vi "FRCts20_Backend_AdministratorInterface.vi"() -> ()   [LabVIEW 2014, in "FRCts20_Backend_TestCode.lvlib"]
uses:
  FRCts20_Backend_TestCode.lvlib
  FRCts20_Backend_Engine.lvlib
  FRCts20_Backend_FGVOperation.ctl
  FRCts20_Backend_DequeueDataOperations.ctl
  FRCts20_Backend_WebMethods.lvlib
  <vilib>/Utility/error.llb/DialogType.ctl
  FRCts20_Backend_IssueDfn.ctl
  FRCts20_Backend_Controls.lvlib
  FRCts20_Backend_TeamDfn.ctl
  FRCts20_Backend_PercTeams.ctl
  FRCts20_Backend_ResDayTotals.ctl
  FRCts20_Backend_ResQuadTotals.ctl
  FRCts20_Backend_OpenQuadTotals.ctl
  FRCts20_Backend_TeamList.ctl
  FRCts20_Backend_IssueTeamList.ctl
  FRCts20_Backend_Team_Info.ctl
  FRCts20_Backend_Note.ctl
  FRCts20_Backend_Note_list.ctl
  FRCts20_Backend_request_info.ctl
panel:
  in  "Tab Control":T1(tab)
  out "Status?":string
  in  "Add Team":bool
  in  "Add Team":T2
  in  "Exit":bool
  in  "Team Number?":u16
  in  "Get Team":bool
  out "Get Team":T2
  out "Key (Return)":string
  out "Message Value (Return)":string
  out "Message (Return)":string
  in  "DeQueue Data":bool
  in  "Key":string
  in  "Message Value":string
  in  "Message Name":string
  in  "Send Meassage":bool
  out "IssueTeamList":T4
  in  "Get Issue Team List":bool
  in  "Get Team List":bool
  out "TeamList":T9
  in  "Get Stats":bool
  out "Issues.Open.QuadTotals":T10
  out "Issues.Open.Total":u16
  out "SoftwareUsage.PercTeams":T11
  out "Issues.Resolved.Total":u16
  out "Issues.Resolved.AvgTimeRes":dbl
  out "Issues.Resolved.QuadTotals":T12
  out "Issues.Resolved.DayTotals":T13
  in  "Exit Run-Time  2":bool
  in  "Edit Exit":bool
  in  "Set Dates":bool
  in  "Competition Start Date":timestamp
  in  "Path to GenerateStats.vi":path=path "C:/FRC Team Service/source/VI Source/FRCts20_Backend_GenerateStats.vi"
  out "Complete?":bool
  # "Run-Time Tools"
  # "Run-Time Tools"
  # "Edit-Time Tools"
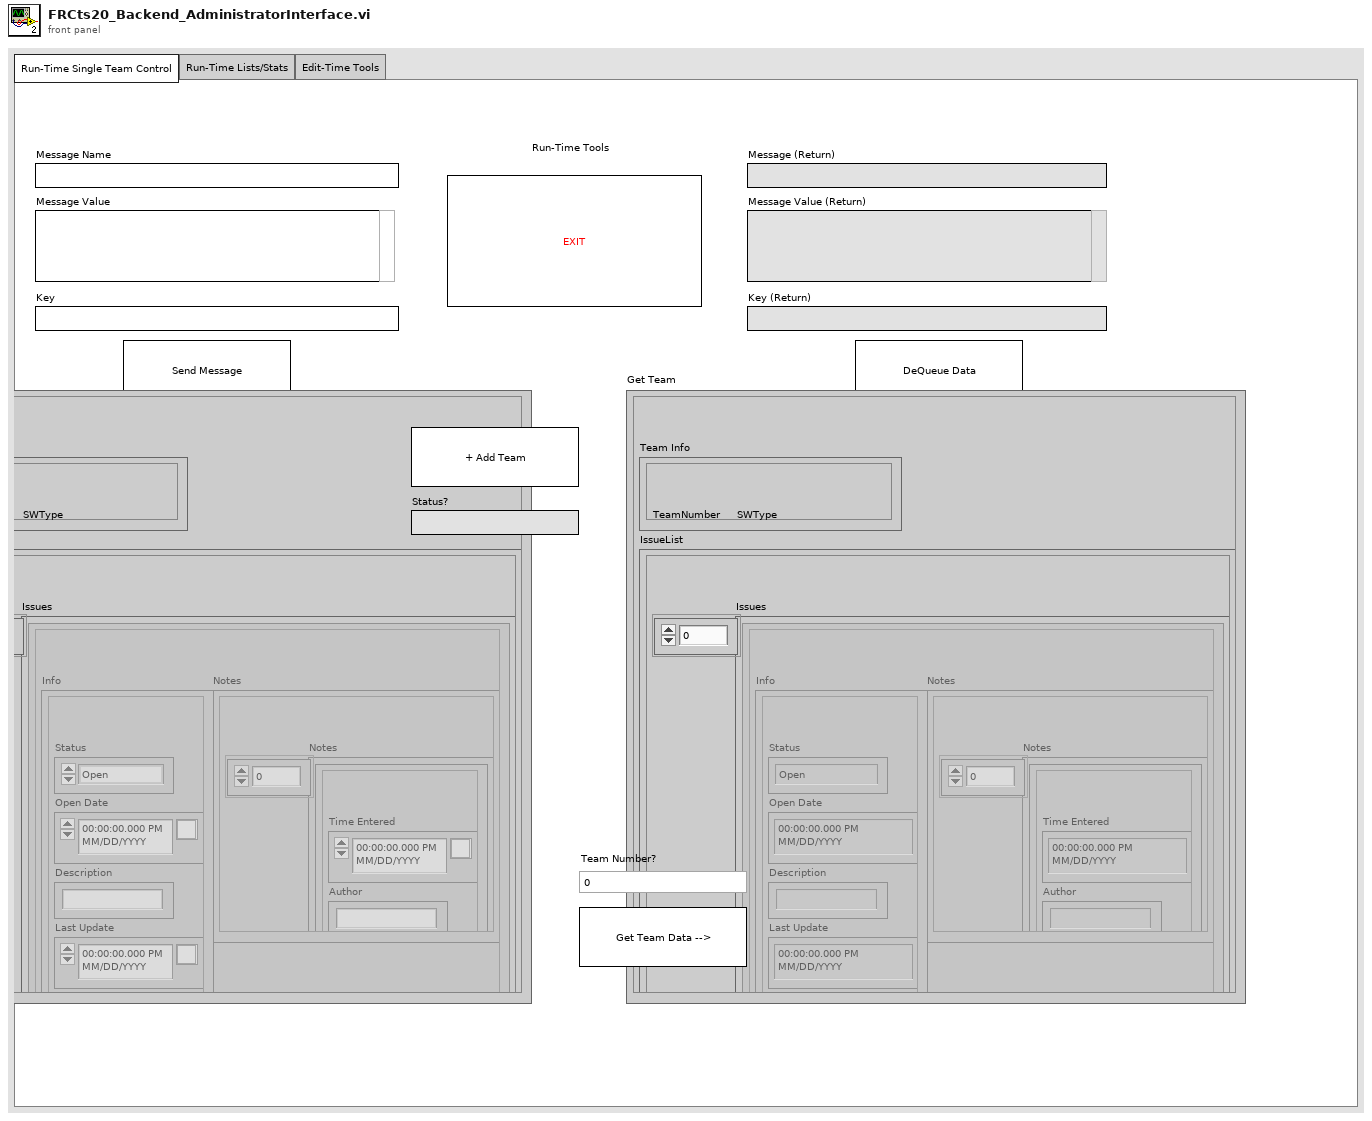
[diagram p1: front panel]
types:
  T1 = enum32{"Run-Time Single Team Control", "Run-Time Lists/Stats", "Edit-Time Tools"}
  T2 = typedef "FRCts20_Backend_Controls.lvlib/FRCts20_Backend_TeamDfn.ctl" = cluster{"Team Info":T3, "IssueList":T4}
  T3 = typedef "FRCts20_Backend_Controls.lvlib/FRCts20_Backend_Team_Info.ctl" = cluster{"TeamNumber":u16, "SWType":string}
  T4 = typedef "FRCts20_Backend_Controls.lvlib/FRCts20_Backend_IssueTeamList.ctl" = cluster{"Issues":T5[]}
  T5 = typedef "FRCts20_Backend_Controls.lvlib/FRCts20_Backend_IssueDfn.ctl" = cluster{"Notes":T6, "Info":T8}
  T6 = typedef "FRCts20_Backend_Controls.lvlib/FRCts20_Backend_Note_list.ctl" = cluster{"Notes":T7[]}
  T7 = typedef "FRCts20_Backend_Controls.lvlib/FRCts20_Backend_Note.ctl" = cluster{"Time Entered":timestamp, "Author":string, "Text":string}
  T8 = typedef "FRCts20_Backend_Controls.lvlib/FRCts20_Backend_request_info.ctl" = cluster{"Status":enum16{"Open", "In Work", "Closed"}, "Open Date":timestamp, "Description":string, "Last Update":timestamp, "Closed Date":timestamp, "Solution Index":i32}
  T9 = typedef "FRCts20_Backend_Controls.lvlib/FRCts20_Backend_TeamList.ctl" = cluster{"Team":cluster{"TeamNumber":u16, "Location":string}[]}
  T10 = typedef "FRCts20_Backend_Controls.lvlib/FRCts20_Backend_OpenQuadTotals.ctl" = cluster{"Quad1":u16, "Quad2":u16, "Quad3":u16, "Quad4":u16}
  T11 = typedef "FRCts20_Backend_Controls.lvlib/FRCts20_Backend_PercTeams.ctl" = cluster{"LabVIEW_Perc":dbl, "C_Cpp_Perc":dbl, "Java_Perc":dbl, "Other_Perc":dbl}
  T12 = typedef "FRCts20_Backend_Controls.lvlib/FRCts20_Backend_ResQuadTotals.ctl" = cluster{"Quad1":u16, "Quad2":u16, "Quad3":u16, "Quad4":u16}
  T13 = typedef "FRCts20_Backend_Controls.lvlib/FRCts20_Backend_ResDayTotals.ctl" = cluster{"Day1":u16, "Day2":u16, "Day3":u16, "Day4":u16}
  T14 = typedef "DialogType.ctl" = u16
  T15 = typedef "FRCts20_Backend_Engine.lvlib/FRCts20_Backend_FGVOperation.ctl" = enum16{"Initialize", "EnqueueMessage", "EnqueueDataReturn", "FlushMessage", "FlushDataReturn"}
  T16 = typedef "FRCts20_Backend_Engine.lvlib/FRCts20_Backend_DequeueDataOperations.ctl" = enum16{"Initialize", "DequeueDataReturn", "GetQueues"}
  T17 = typedef "FRCts20_Backend_Controls.lvlib/FRCts20_Backend_Stats.ctl" = cluster{"SoftwareUsage":T18, "Issues":T20}
  T18 = typedef "FRCts20_Backend_Controls.lvlib/FRCts20_Backend_SoftwareUsage.ctl" = cluster{"NumTeams":T19, "PercTeams":T11}
  T19 = typedef "FRCts20_Backend_Controls.lvlib/FRCts20_Backend_NumTeams.ctl" = cluster{"LabVIEW_Num":u16, "C_Cpp_Num":u16, "Java_Num":u16, "Other_Num":u16}
  T20 = typedef "FRCts20_Backend_Controls.lvlib/FRCts20_Backend_Issues.ctl" = cluster{"Resolved":T21, "Open":T23}
  T21 = typedef "FRCts20_Backend_Controls.lvlib/FRCts20_Backend_Resolved.ctl" = cluster{"Total":u16, "AvgTimeRes":dbl, "PerDayPerQuad":T22, "DayTotals":T13, "QuadTotals":T12}
  T22 = typedef "FRCts20_Backend_Controls.lvlib/FRCts20_Backend_ResPerDayPerQuad.ctl" = cluster{"Day1Quad1":u16, "Day1Quad2":u16, "Day1Quad3":u16, "Day1Quad4":u16, "Day2Quad1":u16, "Day2Quad2":u16, "Day2Quad3":u16, "Day2Quad4":u16, "Day3Quad1":u16, "Day3Quad2":u16, "Day3Quad3":u16, "Day3Quad4":u16, "Day4Quad1":u16, "Day4Quad2":u16, "Day4Quad3":u16, "Day4Quad4":u16}
  T23 = typedef "FRCts20_Backend_Controls.lvlib/FRCts20_Backend_Open.ctl" = cluster{"Total":u16, "QuadTotals":T10}
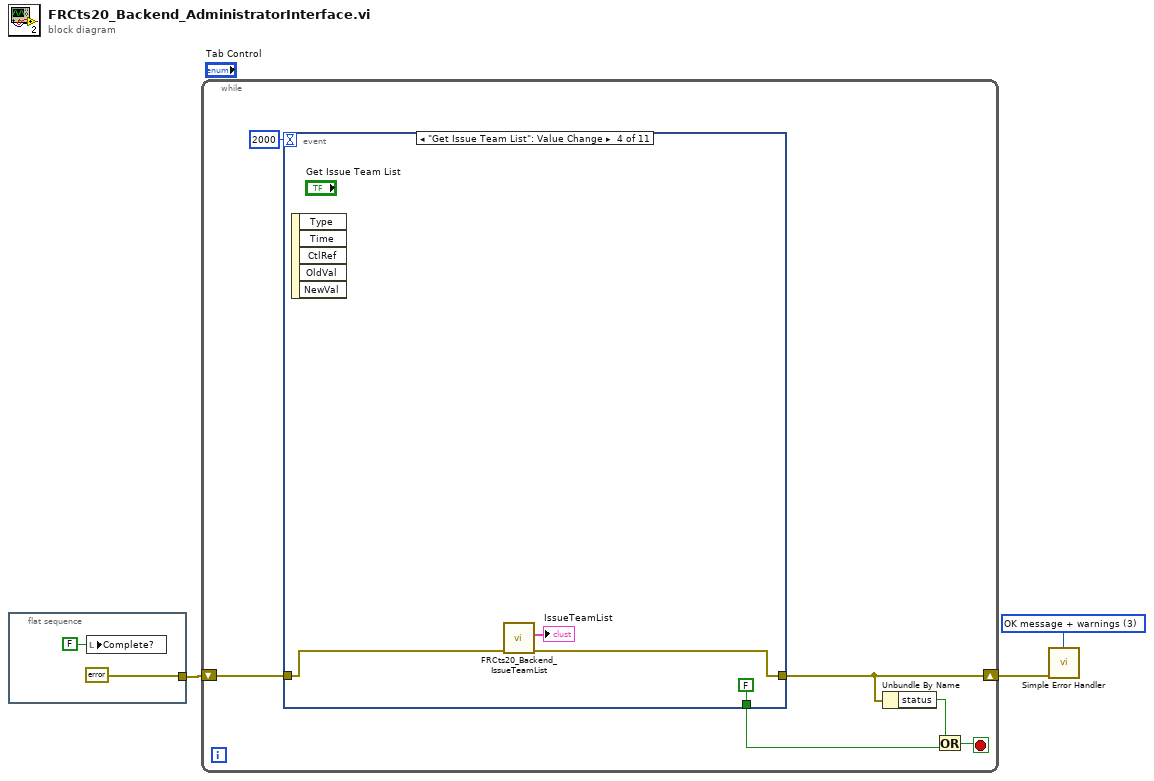
[diagram p0: block diagram]
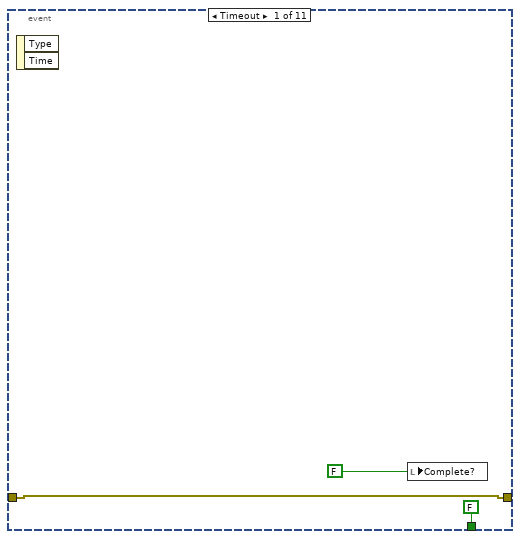
[diagram p2: hidden frame]
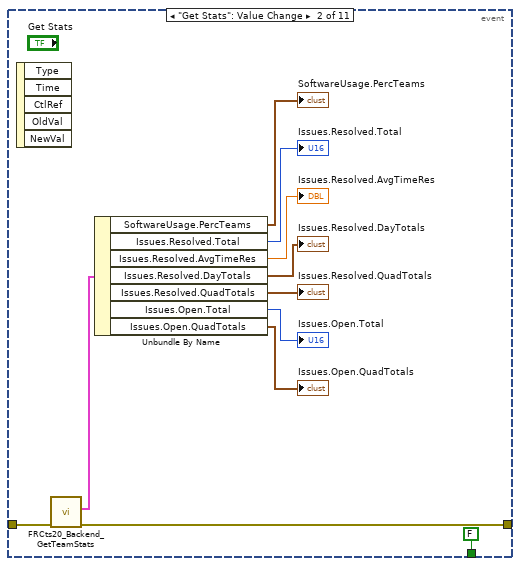
[diagram p3: hidden frame]
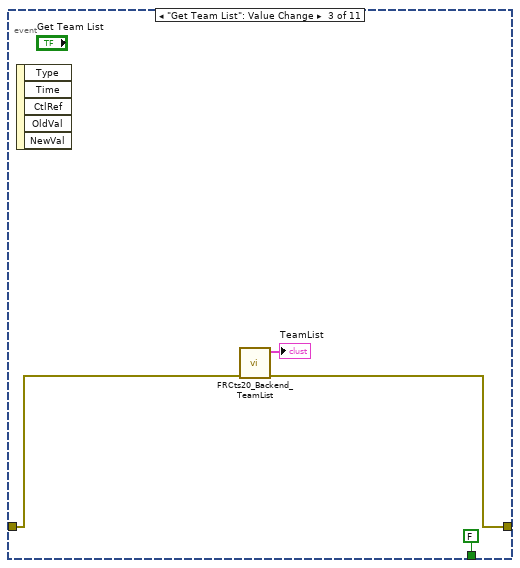
[diagram p4: hidden frame]
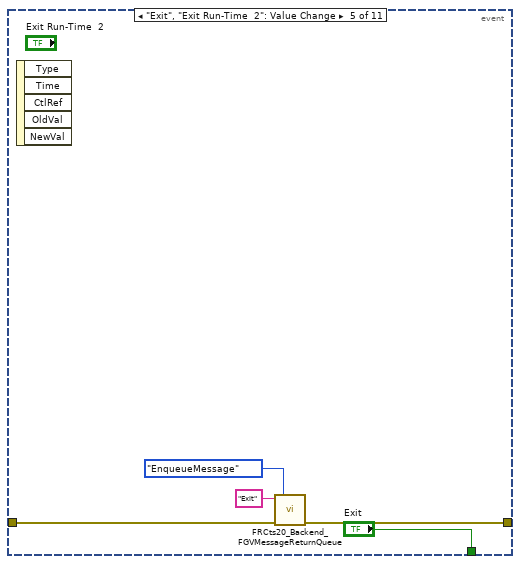
[diagram p5: hidden frame]
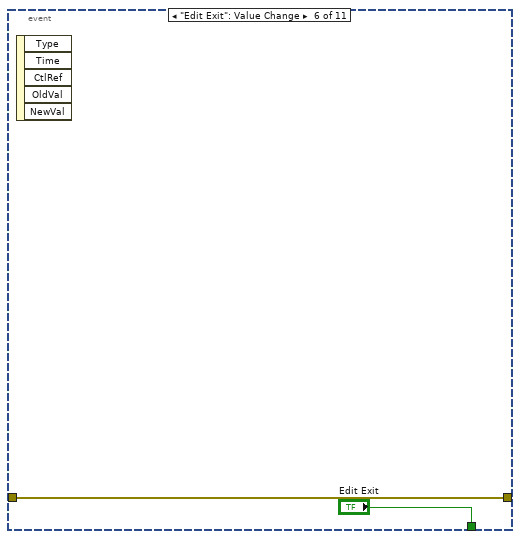
[diagram p6: hidden frame]
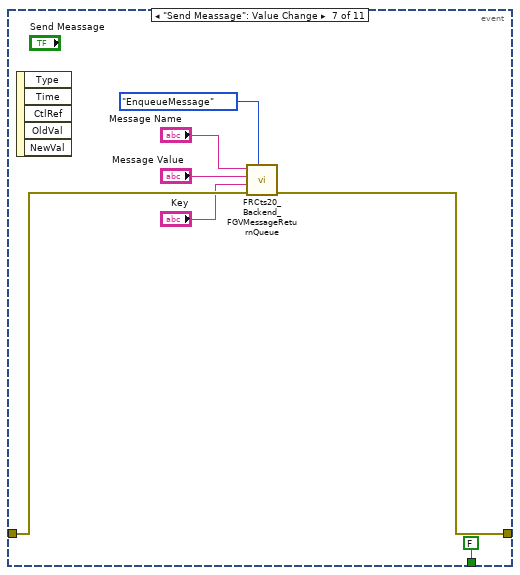
[diagram p7: hidden frame]
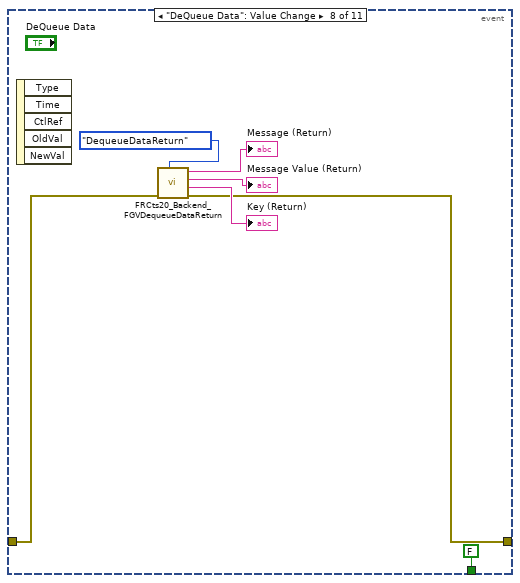
[diagram p8: hidden frame]
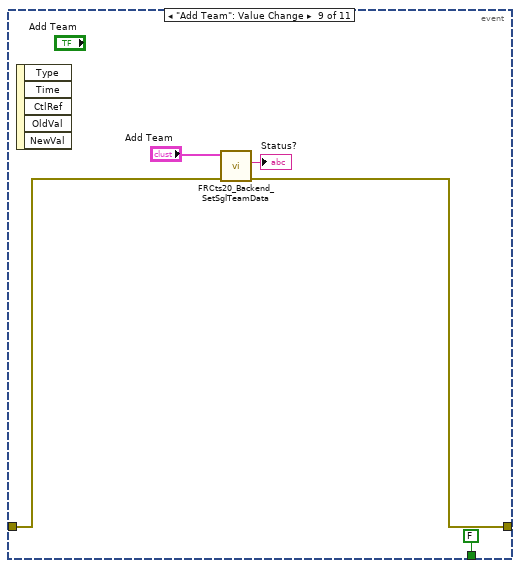
[diagram p9: hidden frame]
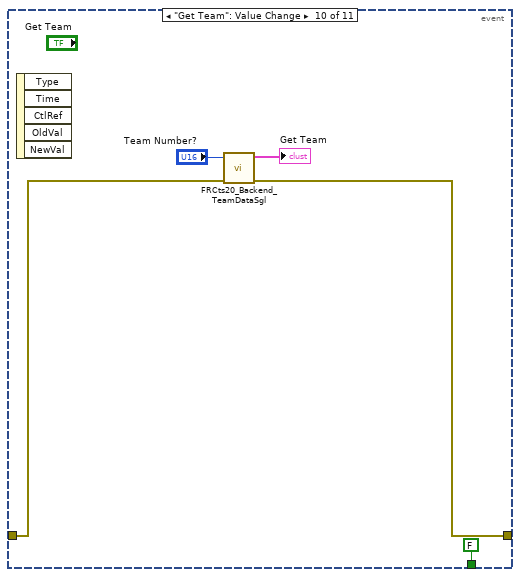
[diagram p10: hidden frame]
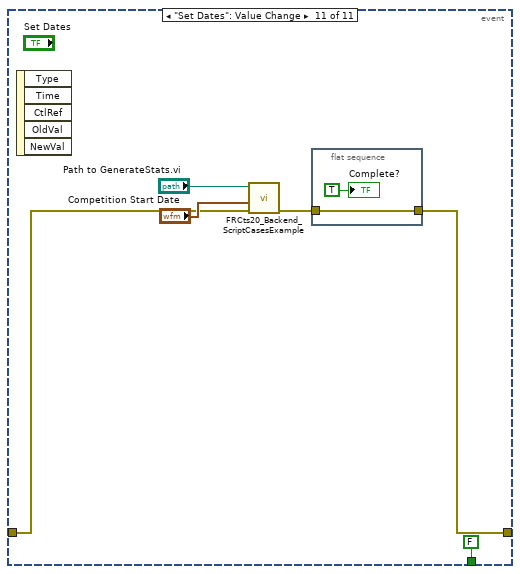
[diagram p11: hidden frame]
diagram:
  w2 = T14 3 items=["no dialog", "OK message", "continue or stop message", "OK message + warnings", "continue/stop + warnings"] ("type of dialog (OK msg:1)")
  n1 = flat-sequence {
    tunnel: [errorcluster {"status"=FALSE, "code"=0, "source"=""} ("error in (no error)")] -> w1
    frame #0 {
      n2 = local write "Complete?"(FALSE ("Complete?")) -> ()
    }
  }
  n3 = while {
    shift-right: [w9] -> w3
    shift-left: w1 -> [w10]
    stop <- w8 stop-if-true
    n4 = event shown="[3] \"Get Issue Team List\": Value Change" {
      selector: _ -> [_ _ _ _ _ _ _ _ _ _ _]
      dyn-events: _ -> [_ _ _ _ _ _ _ _ _ _ _]
      timeout: 2000 -> [_ _ _ _ _ _ _ _ _ _ _]
      tunnel: w10 -> [w13 w25 w29 w33 w37 w39 w47 w54 w59 w64 w68]
      tunnel: [w13 w24 w28 w32 w36 w39 w42 w49 w57 w63 w65] -> w9
      tunnel: [FALSE ("Exit") FALSE ("Exit") FALSE ("Exit") FALSE ("Exit") "Exit" "Edit Exit" FALSE ("Exit") FALSE ("Exit") FALSE ("Exit") FALSE ("Exit") FALSE ("Exit")] -> w6
      event Timeout {
        n5 = event-data() -> ()  [unwired: 1 in, 2 out]
        n6 = local write "Complete?"(FALSE ("Complete?")) -> ()
      }
      event "Get Stats": Value Change {
        n7 = event-data() -> ()  [unwired: 1 in, 5 out]
        n8 = call "FRCts20_Backend_GetTeamStats.vi"("error in (no error)"=w25) -> ("error out"=w24:errorcluster, "Stats"=w23:T17)  [unwired: 9 in]
        n9 = Unbundle By Name(w23) -> ("SoftwareUsage.PercTeams"=→"SoftwareUsage.PercTeams":T11, "Issues.Resolved.Total"=→"Issues.Resolved.Total":u16, "Issues.Resolved.AvgTimeRes"=→"Issues.Resolved.AvgTimeRes":dbl, "Issues.Resolved.DayTotals"=→"Issues.Resolved.DayTotals":T13, "Issues.Resolved.QuadTotals"=→"Issues.Resolved.QuadTotals":T12, "Issues.Open.Total"=→"Issues.Open.Total":u16, "Issues.Open.QuadTotals"=→"Issues.Open.QuadTotals":T10)
      }
      event "Get Team List": Value Change {
        n10 = event-data() -> ()  [unwired: 1 in, 5 out]
        n11 = call "FRCts20_Backend_TeamList.vi"("error in (no error)"=w29) -> ("error out"=w28:errorcluster, "TeamList"=→"TeamList":T9)  [unwired: 9 in]
      }
      event "Get Issue Team List": Value Change {
        n12 = event-data() -> ()  [unwired: 1 in, 5 out]
        n13 = call "FRCts20_Backend_IssueTeamList.vi"("error in (no error)"=w33) -> ("error out"=w32:errorcluster, "IssueTeamList"=→"IssueTeamList":T4)  [unwired: 9 in]
      }
      event "Exit", "Exit Run-Time  2": Value Change {
        n14 = event-data() -> ()  [unwired: 1 in, 5 out]
        n15 = call "FRCts20_Backend_FGVMessageReturnQueue.vi"("Operation"=FRCts20_Backend_FGVOperation."EnqueueMessage", "error in (no error)"=w37, "Message Name"="Exit") -> ("error out"=w36:errorcluster)  [unwired: 5 in, 1 out]
      }
      event "Edit Exit": Value Change {
        n16 = event-data() -> ()  [unwired: 1 in, 5 out]
      }
      event "Send Meassage": Value Change {
        n17 = event-data() -> ()  [unwired: 1 in, 5 out]
        n18 = call "FRCts20_Backend_FGVMessageReturnQueue.vi"("Operation"=FRCts20_Backend_FGVOperation."EnqueueMessage", "error in (no error)"=w47, "Key"="Key", "Message Value"="Message Value", "Message Name"="Message Name") -> ("error out"=w42:errorcluster)  [unwired: 3 in, 1 out]
      }
      event "DeQueue Data": Value Change {
        n19 = event-data() -> ()  [unwired: 1 in, 5 out]
        n20 = call "FRCts20_Backend_FGVDequeueDataReturn.vi"("Operation"=FRCts20_Backend_DequeueDataOperations."DequeueDataReturn", "error in (no error)"=w54) -> ("error out"=w49:errorcluster, "Key"=→"Key (Return)":string, "Message Value"=→"Message Value (Return)":string, "Message Name"=→"Message (Return)":string)  [unwired: 5 in, 1 out]
      }
      event "Add Team": Value Change {
        n21 = event-data() -> ()  [unwired: 1 in, 5 out]
        n22 = call "FRCts20_Backend_SetSglTeamData.vi"("error in (no error)"=w59, "Team"="Add Team") -> ("error out"=w57:errorcluster, "Status?"=→"Status?":string)  [unwired: 8 in]
      }
      event "Get Team": Value Change {
        n23 = event-data() -> ()  [unwired: 1 in, 5 out]
        n24 = call "FRCts20_Backend_TeamDataSgl.vi"("error in (no error)"=w64, "TeamNum"="Team Number?") -> ("error out"=w63:errorcluster, "TeamDataOut"=→"Get Team":T2)  [unwired: 8 in]
      }
      event "Set Dates": Value Change {
        n25 = event-data() -> ()  [unwired: 1 in, 5 out]
        n26 = call "FRCts20_Backend_ScriptCasesExample.vi"("error in (no error)"=w68, "Competition Start Date"="Competition Start Date", "Path to Stats"="Path to GenerateStats.vi") -> ("error out"=w66:errorcluster)  [unwired: 8 in]
        n27 = flat-sequence {
          tunnel: w66 -> [w71]
          tunnel: [w71] -> w65
          frame #0 {
            "Complete?" <- TRUE ("Complete?")
          }
        }
      }
    }
    n28 = Unbundle By Name(w9) -> ("status"=w7:bool)
    n29 = Or(x=w7, y=w6) -> (x .or. y?=w8:bool)
  }
  n30 = call <vilib>:"Simple Error Handler.vi"("type of dialog (OK msg:1)"=w2, "error in (no error)"=w3) -> ()  [unwired: 3 in, 5 out]
